vi "Equals Abstract Handler.vi"(10 "Controller Event Fire Handler":refnum<class "Abstract Event Handler for Controller.lvclass">) -> (2 "Is Abstract Event Handler":bool)   [LabVIEW 2017, in "Event Actors.lvlib" / "Abstract Event Handler for Controller.lvclass"]
uses:
  Abstract Event Handler for Controller.lvclass
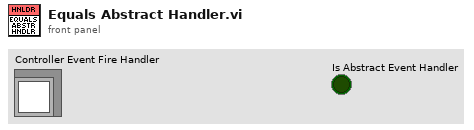
[diagram p1: front panel]
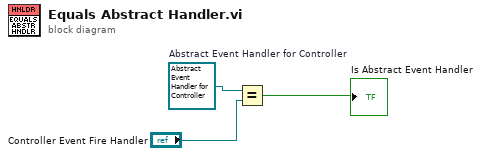
[diagram p0: block diagram]
diagram:
  w3 = refnum<class "Abstract Event Handler for Controller.lvclass"> refnum  # Abstract Event Handler for Controller
  n1 = Equal?(x=w3, y="Controller Event Fire Handler") -> (x = y?=→"Is Abstract Event Handler":bool)
